vi "Load Scale.vi"(8 "err in":errorcluster caption="エラー入力（エラーなし）", 11 "WaveformGraph入力":refnum<vi>) -> (0 "err out":errorcluster caption="エラー出力")   [LabVIEW 2014]
uses:
  ScaleParam.ctl
  <vilib>/Utility/miscctls.llb/LVRangeTypeDef.ctl
  PlotParam.ctl
  <vilib>/Utility/xml.llb/Read From XML File(string).vi
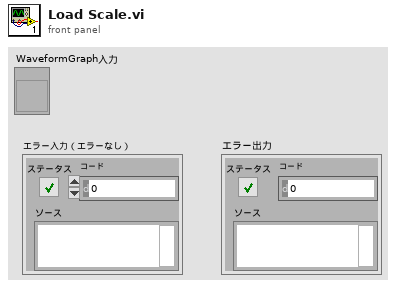
[diagram p1: front panel]
types:
  T1 = typedef "PlotParam.ctl" = cluster{"Plot Color":u32, "Point Style":u8, "Line Width":u8, "Visible?":bool, "XScaleIdx":u32, "YScaleIdx":u32}
  T2 = typedef "ScaleParam.ctl" = cluster{"NameLbl.Text":string, "UnitLabel.Text":string, "Range":T3}
  T3 = typedef "LVRangeTypeDef.ctl" = cluster{"Minimum":dbl, "Maximum":dbl, "Increment":dbl, "Minor Increment":dbl, "Start":dbl}
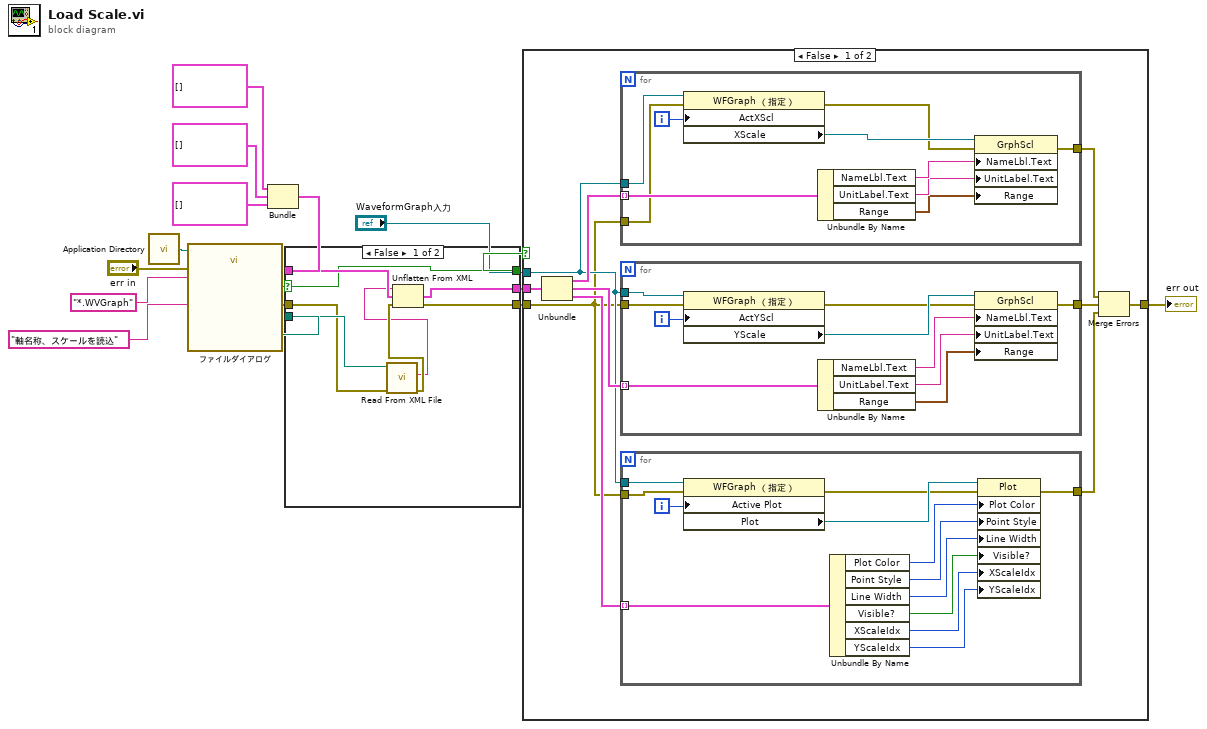
[diagram p0: block diagram]
diagram:
  n1 = call <vilib>:"Application Directory.vi"() -> ("Application Directory"=w15:path)
  n2 = call "ファイルダイアログ"("start path"=w15, "prompt"="軸名称、スケールを読込", "error in"="err in", "pattern (all files)"="*.WVGraph") -> ("selected path"=w10:path, "cancelled"=w12:bool, "error out"=w11:errorcluster)  [unwired: 8 in, 1 out]
  n3 = Bundle(T2[] [], T2[] [], T1[] []) -> (w16:cluster{T2[], T2[], T1[]})  [unwired: 1 in]
  n4 = case shown="FALSE" w12 {
    selector: w12 -> [w21 w25]
    tunnel: [w22 w26] -> w8
    tunnel: w16 -> [w24 _]
    tunnel: w11 -> [w19 w26]
    tunnel: w10 -> [w20 _]
    tunnel: [w23 _] -> w9
    tunnel: [w21 w25] -> w6
    frame False {
      n5 = call-poly <vilib>:"Read From XML File.vi"("error in (no error)"=w19, "XML File Path"=w20) -> ("error out"=w18:errorcluster, "XML Elements"=w17:string)  [unwired: 7 in, 1 out]
      n6 = Unflatten From XML(xml string=w17, type=w24, error in (no error)=w18) -> (value=w23:cluster{T2[], T2[], T1[]}, error out=w22:errorcluster)
    }
    frame True {
    }
  }
  n7 = case shown="FALSE" w6 {
    tunnel: w9 -> [w36 _]
    tunnel: "WaveformGraph入力" -> [w30 _]
    tunnel: w8 -> [w28 w70]
    tunnel: [w33 w70] -> w7
    frame False {
      n8 = Unbundle(w36) -> (w32:T2[], w31:T2[], w29:T1[])
      n9 = for {
        tunnel: w32 -> [w66] mode=indexing
        tunnel: w30 -> [w68]
        tunnel: w28 -> [w62]
        tunnel: [w60] -> w35
        i -> [w69]
        n10 = property class="WFGraph （指定）"(reference=w68, error in=w62, "ActXScl"=w69) -> (error out=w61:errorcluster, "XScale"=w67:refnum<vi>)  [unwired: 1 out]
        n11 = Unbundle By Name(w66) -> ("NameLbl.Text"=w65:string, "UnitLabel.Text"=w64:string, "Range"=w63:T3)
        n12 = property class="GrphScl"(reference=w67, error in=w61, "NameLbl.Text"=w65, "UnitLabel.Text"=w64, "Range"=w63) -> (error out=w60:errorcluster)  [unwired: 1 out]
      }
      n13 = for {
        tunnel: w31 -> [w56] mode=indexing
        tunnel: w30 -> [w58]
        tunnel: w28 -> [w52]
        tunnel: [w50] -> w34
        i -> [w59]
        n14 = property class="WFGraph （指定）"(reference=w58, error in=w52, "ActYScl"=w59) -> (error out=w51:errorcluster, "YScale"=w57:refnum<vi>)  [unwired: 1 out]
        n15 = Unbundle By Name(w56) -> ("NameLbl.Text"=w55:string, "UnitLabel.Text"=w54:string, "Range"=w53:T3)
        n16 = property class="GrphScl"(reference=w57, error in=w51, "NameLbl.Text"=w55, "UnitLabel.Text"=w54, "Range"=w53) -> (error out=w50:errorcluster)  [unwired: 1 out]
      }
      n17 = for {
        tunnel: w29 -> [w46] mode=indexing
        tunnel: w30 -> [w48]
        tunnel: w28 -> [w45]
        tunnel: [w43] -> w27
        i -> [w49]
        n18 = property class="WFGraph （指定）"(reference=w48, error in=w45, "Active Plot"=w49) -> (error out=w44:errorcluster, "Plot"=w47:refnum<vi>)  [unwired: 1 out]
        n19 = Unbundle By Name(w46) -> ("Plot Color"=w42:u32, "Point Style"=w41:u8, "Line Width"=w40:u8, "Visible?"=w39:bool, "XScaleIdx"=w38:u32, "YScaleIdx"=w37:u32)
        n20 = property class="Plot"(reference=w47, error in=w44, "Plot Color"=w42, "Point Style"=w41, "Line Width"=w40, "Visible?"=w39, "XScaleIdx"=w38, "YScaleIdx"=w37) -> (error out=w43:errorcluster)  [unwired: 1 out]
      }
      n21 = Merge Errors(w35, w34, w27) -> (w33:errorcluster)
    }
    frame True {
    }
  }
  "err out" <- w7
